vi "Validate Reference by GUID.vi"(8 "error in":errorcluster, 9 "name":string, 10 "guid":string, 11 "slsc switch item in":T1 format="%.0x") -> (0 "error out":errorcluster, 3 "slsc switch item out":T1 format="%.0x")   [LabVIEW 2020, in "SLSC Switch Scripting.lvlib"]
uses:
  SLSC Switch Scripting.lvlib
  <vilib>/NI VeriStand/Custom Device API/Custom Device Item Ref.ctl
  NationalInstruments.VeriStand.SystemDefinitionAPI
  <vilib>/NI VeriStand/Custom Device API/Custom Device API.lvlib
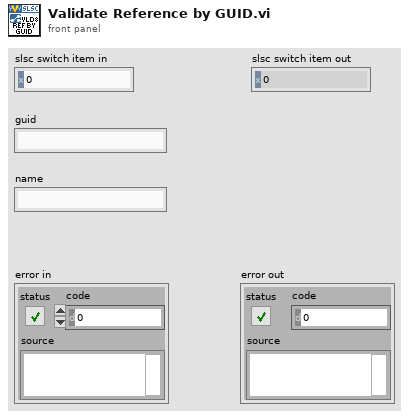
[diagram p1: front panel]
types:
  T1 = typedef "Custom Device API.lvlib/Custom Device Item Ref.ctl" = u64
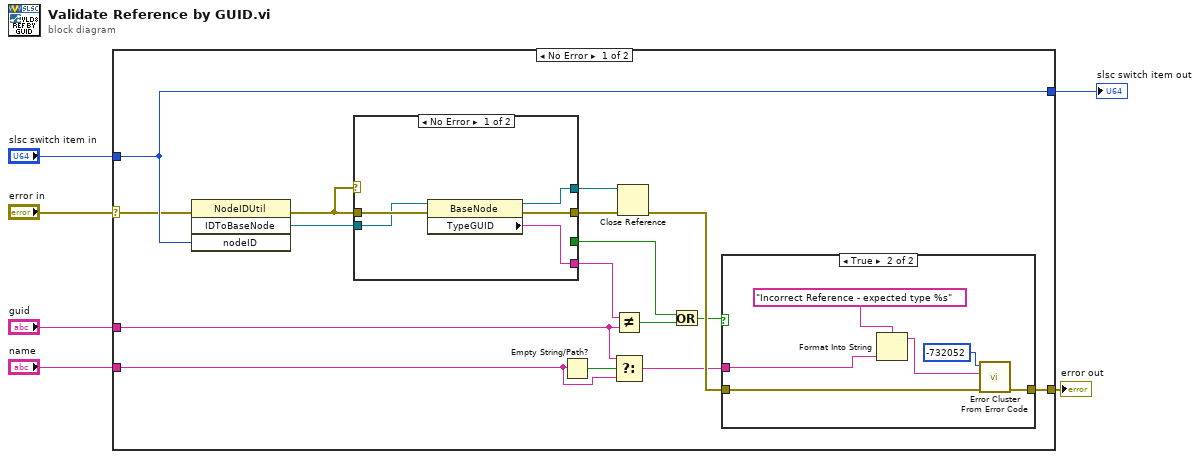
[diagram p0: block diagram]
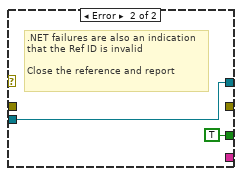
[diagram p2: hidden frame]
diagram:
  n1 = case shown="No Error" "error in" {
    selector: "error in" -> [w11 w37]
    tunnel: [w17 w37] -> w6
    tunnel: "guid" -> [w7 _]
    tunnel: "slsc switch item in" -> [w12 w38]
    tunnel: [w12 w38] -> w3
    tunnel: "name" -> [w9 _]
    frame No Error {
      n2 = invoke class="NodeIDUtil" method="IDToBaseNode"(error in=w11, "nodeID"=w12) -> (error out=w16:errorcluster, "IDToBaseNode"=w19:refnum<k24>)  [unwired: 2 in, 2 out]
      n3 = case shown="No Error" w16 {
        tunnel: [w27 _] -> w22
        tunnel: [w26 _] -> w21
        tunnel: [w25 w29] -> w20
        tunnel: w16 -> [w24 _]
        tunnel: w19 -> [w23 w29]
        tunnel: [_ TRUE] -> w14
        frame No Error {
          n4 = property class="BaseNode"(reference=w23, error in=w24) -> (reference out=w25:refnum<k24>, error out=w26:errorcluster, "TypeGUID"=w27:string)
        }
        frame Error {
          # ".NET failures are also an indication\nthat the Ref ID is invalid\n\nClose the reference and report"
        }
      }
      n5 = Empty String/Path?(string/path=w9) -> (empty?=w10:bool)
      n6 = Not Equal?(x=w22, y=w7) -> (x != y?=w13:bool)
      n7 = Select(t=w7, s=w10, f=w9) -> (s? t:f=w8:string)
      n8 = Close Reference(reference=w20, error in (no error)=w21) -> (error out=w18:errorcluster)
      n9 = Or(x=w14, y=w13) -> (x .or. y?=w15:bool)
      n10 = case shown="True" w15 {
        tunnel: w18 -> [w30 w35]
        tunnel: [w30 w34] -> w17
        tunnel: w8 -> [_ w31]
        frame False {
        }
        frame True {
          n11 = Format Into String(format string="Incorrect Reference - expected type %s" ("error message (\"\")"), w31) -> (resulting string=w32:string)  [unwired: 2 in, 1 out]
          n12 = call <vilib>:"Error Cluster From Error Code.vi"("error in (no error)"=w35, "error message (\"\")"=w32, "error code (0)"=-732052) -> ("error out"=w34:errorcluster)  [unwired: 6 in]
        }
      }
    }
    frame Error {
    }
  }
  "error out" <- w6
  "slsc switch item out" <- w3
